vi "ElapsedAndRemainingTime.vi"(7 "Time period target":i32 caption="Time period target (0) [ms]" min=0, 11 "Error in":errorcluster caption="Error in (no error)", 12 "Start time in":i32 caption="Start time in (0) [ms]" min=0) -> (8 "Remaining time":i32 caption="Remaining time [ms]", 10 "Elapsed time":i32 caption="Elapsed time [ms]", 13 "This start time out":i32 caption="This start time out [ms]", 14 "Start time out":i32 caption="Start time out [ms]", 15 "Error out":errorcluster)   [LabVIEW 2017, in "GPTiming.lvlib"]
doc: "THIS FUNCTION IS DEPRECATED AND SHOULD BE REPLACED WITH THE ElapsedTime OR RemainingTime FUNCTION THAT REPLACES IT.\n\n**************************************************\n\nAt the time this function is called (\"Now\"), these values will be calculated;\n\n1) <B>Remaining time</B> from a comparison between <B>Start time in</B> and <B>Time period target</B>, and\n2) <B>Elapsed time</B> since <B>Start time in</B>.\n\n<B>Remaining time</B> will count down until reaching zero, at which point it's latched at zero. The internal counter is an U32, so <B>Remaining time</B> remains reliably latched at zero for slightly more than 1193 hours after <B>Start time in</B> (2^32-1 ms).\n\n<B>Elapsed time</B> will continue counting up even after <B>Remaining time</B> is latched at zero, and will remain reliable for a bit more than 596 hours after <B>Start time in</B> (2^31-1 ms).\n\nSet <B>Start time in</B> to zero (or leave it unwired) to get the current time returned in <B>Start time out</B>. This way you prime the function for the first iteration in a loop. Afterwards you just daisychain <B>Start time out</B> to <B>Start time in</B> of the next ElapsedAndRemainingTime function (or back to the same ElapsedAndRemainingTime function via a shift register or feedback node).\n\n<B>This start time out</B> will always be the start time of the VI instance. Wire this to <B>Start time in</B> of the next ElapsedAndRemainingTime function to calculate <B>Elapsed time</B> of the code between them.\n\n<B>Common use cases:</B>\n\nFacilitate timeout in a variable cycle-time loop:\nPlace a single ElapsedAndRemainingTime function at the start of the cycle, maintain the start time in a shift register (initialized to zero), wire your timeout value to <B>Time period target</B>, and end the loop when <B>Remaining time</B> reaches zero.\n\nMeasure execution time of one or more sections of code:\nIf you want to measure the execution time of a section of code, you wrap the code section with ElapsedAndRemainingTime functions, daisy chain <B>Start time out</B> to <B>Start time in</B>, and read the execution time from the <B>Elapsed time</B> output of the last ElapsedAndRemainingTime function.\n\nThis VI is inlined. <B>Error in</B> is wired straight through to <B>Error out</B> to enable optional data-flow dependency (offering control of when \"Now\" is obtained).\n\nSteen Schmidt\nGPower\n1/1 2013"
uses:
  GPTiming.lvlib
panel:
  # "Copyright © 2013\nGPower\nSee enclosed license file for terms and conditions"
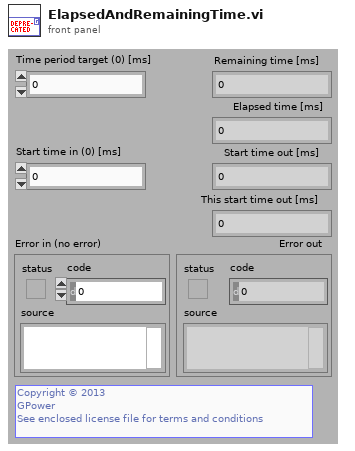
[diagram p1: front panel]
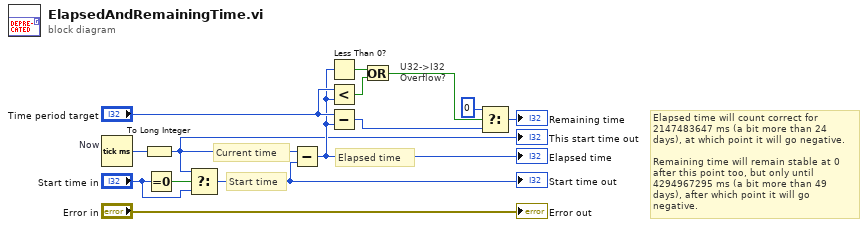
[diagram p0: block diagram]
diagram:
  # "Elapsed time will count correct for 2147483647 ms (a bit more than 24 days), at which point it will go negative.\n\nRemaining time will remain stable at 0 after this point too, but only until 4294967295 ms (a bit more than 49 days), after which point it will go negative."
  # "Elapsed time"
  # "U32->I32\nOverflow?"
  # "Current time"
  # "Start time"
  n1 = Tick Count (ms) "Now"() -> (millisecond timer value=w9:u32)
  n2 = To Long Integer(number=w9) -> (32bit integer=w1:i32)
  "This start time out" <- w1
  n3 = Equal To 0?(x="Start time in") -> (x = 0?=w14:bool)
  n4 = Select(t=w1, s=w14, f="Start time in") -> (s? t:f=w8:i32)
  "Start time out" <- w8
  n5 = Subtract(x=w1, y=w8) -> (x-y=w5:i32)
  "Elapsed time" <- w5
  n6 = Less Than 0?(x=w5) -> (x < 0?=w4:bool)
  n7 = Less?(x="Time period target", y=w5) -> (x < y?=w3:bool)
  n8 = Subtract(x="Time period target", y=w5) -> (x-y=w6:i32)
  n9 = Or(x=w4, y=w3) -> (x .or. y?=w2:bool)
  n10 = Select(t=0, s=w2, f=w6) -> (s? t:f=→"Remaining time":i32)
  "Error out" <- "Error in"
